vi "Last Ack.vi"(7 "Sender":refnum<class "Sender.lvclass">, 10 "Actor":refnum<class "Actor.lvclass">, 11 "Last Ack in":refnum<class "Last Ack.lvclass">) -> (3 "Last Ack out":refnum<class "Last Ack.lvclass">)   [LabVIEW 2020, in "jettl.lvlib" / "Last Ack Msg.lvlib" / "Last Ack.lvclass"]
uses:
  Last Ack.lvclass
  Actor/Actor/Actor.lvclass
  Sender/Sender/Sender.lvclass
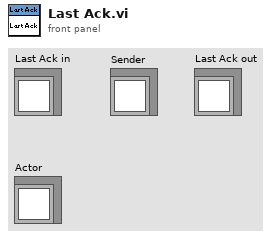
[diagram p1: front panel]
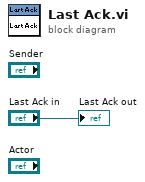
[diagram p0: block diagram]
diagram:
  "Last Ack out" <- "Last Ack in"
